vi "Get Input Array Index.vi"(8 "error in (no error)":errorcluster, 11 "Array in":refnum<vi>) -> (0 "error out":errorcluster, 2 "Index":u32, 3 "Array out":refnum<vi>)   [LabVIEW 2015, in "CallVIStep.lvclass"]
uses:
  CallVIStep.lvclass
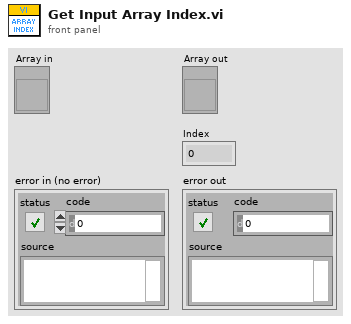
[diagram p1: front panel]
types:
  T1 = typedef "LVRectTypeDef.ctl" = cluster{"Left":i16, "Top":i16, "Right":i16, "Bottom":i16}
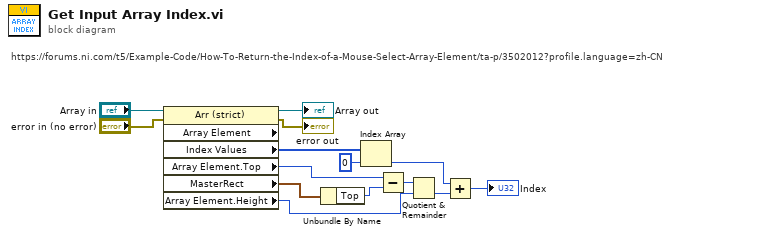
[diagram p0: block diagram]
diagram:
  # "https://forums.ni.com/t5/Example-Code/How-To-Return-the-Index-of-a-Mouse-Select-Array-Element/ta-p/3502012?profile.language=zh-CN"
  n1 = property class="Arr (strict)" props=["Array Element", "Index Values", "Array Element", "Top", "MasterRect", "Array Element", "Height"](reference="Array in", error in="error in (no error)") -> (reference out=→"Array out":refnum<vi>, error out=→"error out":errorcluster, "Index Values"=w14:u32[], "Array Element.Top"=w13:i32, "MasterRect"=w12:T1, "Array Element.Height"=w9:u32)  [unwired: 1 out]
  n2 = Unbundle By Name(w12) -> ("Top"=w11:i16)
  n3 = Index Array(array=w14, index=0) -> (element=w7:u32)
  n4 = Subtract(x=w13, y=w11) -> (x-y=w10:i32)
  n5 = Quotient & Remainder(x=w10, y=w9) -> (floor(x/y)=w6:u32)  [unwired: 1 out]
  n6 = Add(x=w7, y=w6) -> (x+y=→"Index":u32)
